vi "run.vi"(8 "error in (no error)":errorcluster) -> (0 "error out":errorcluster)   [LabVIEW 2011]
panel:
  in  "Path":path=path "C:/Users/Public/Documents/National Instruments/CNC/G-code interperter/G-code.txt"
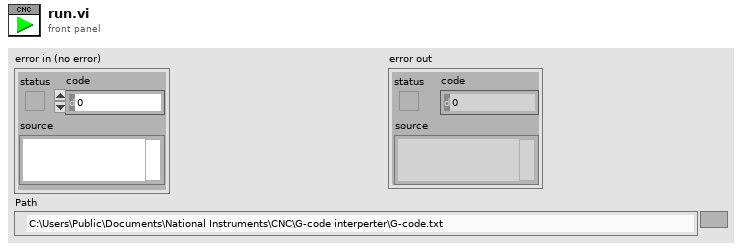
[diagram p1: front panel]
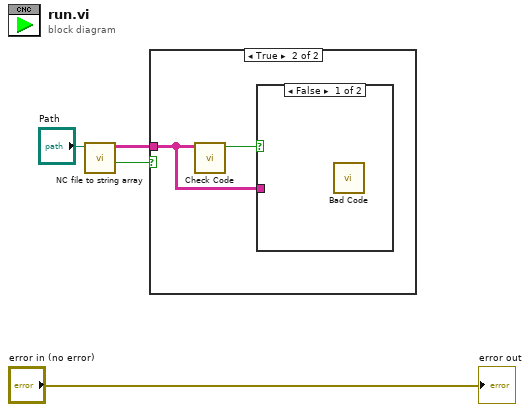
[diagram p0: block diagram]
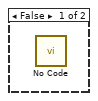
[diagram p2: hidden frame]
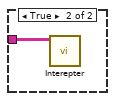
[diagram p3: hidden frame]
diagram:
  n1 = call "NC file to string array.vi"("Path"="Path") -> ("Has Code?"=w4:bool, "Code"=w3:string[][])  [unwired: 9 in]
  n2 = case shown="True" w4 {
    tunnel: w3 -> [_ w5]
    frame False {
      n3 = call "No Code.vi"() -> ()  [unwired: 12 in]
    }
    frame True {
      n4 = call "Check Code.vi"("Code"=w5) -> ("Code Good"=w6:bool)  [unwired: 10 in]
      n5 = case shown="False" w6 {
        tunnel: w5 -> [_ w7]
        frame False {
          n6 = call "Bad Code.vi"() -> ()  [unwired: 12 in]
        }
        frame True {
          n7 = call "Interepter.vi"("Array"=w7) -> ()  [unwired: 11 in]
        }
      }
    }
  }
  "error out" <- "error in (no error)"
